vi "TestDigitizer.vi"() -> ()   [LabVIEW 2018]
uses:
  <extravilib>/ChannelInstances/Tag-c(t'DigitizerInfo.ctl',bool).lvlib
  <vilib>/userdefined/High Color/nirio_resource_hc.ctl
  D:/HardwareRevamp/AcustoXv2/Controls/DigitizerInfo.ctl
panel:
  in  "Digitizer ID":tag
  out "TIS Configured?":bool
  out "Clocking Option Configured?":bool
  out "Default Configured?":bool
  in  "Trigger Type":enum8{"Software", "Data Edge"}(ring)
  in  "Record Size (Samples)":u32=1024
  in  "Trigger Level (V)":dbl
  in  "Delay after Trigger (us)":dbl
  in  "Sampling Rate (Fs)":dbl=400000000.0 format="%#_6p"
  in  "Setup Digitizer":bool
  out "Digitizer Configured?":bool
  out "Digitizer Info":T1
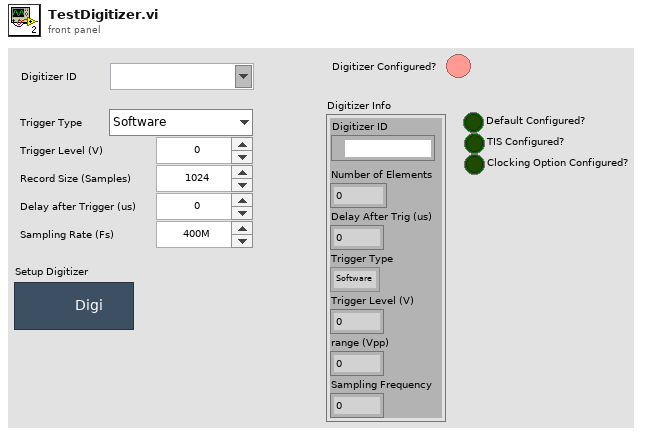
[diagram p1: front panel]
types:
  T1 = typedef "DigitizerInfo.ctl" = cluster{"Digitizer ID":T2, "Number of Elements":u16, "Delay After Trig (us)":dbl, "Trigger Type":enum8{"Software", "Data Edge"}, "Trigger Level (V)":dbl, "range (Vpp)":dbl, "Sampling Frequency":dbl}
  T2 = typedef "nirio_resource_hc.ctl" = tag
  T3 = typedef "Tag-c(t'DigitizerInfo.ctl',bool).lvlib/))Channel.ctl" = refnum<queue>
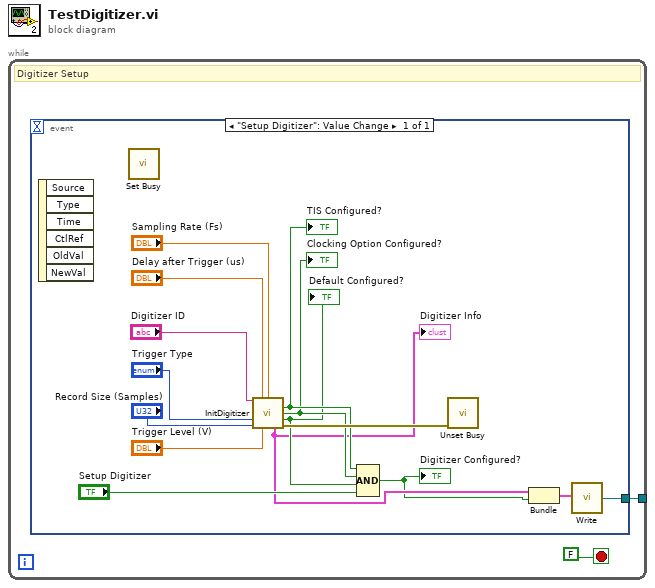
[diagram p0: block diagram]
diagram:
  n1 = while {
    tunnel: [w1] -> _
    stop <- FALSE stop-if-true
    # "Digitizer Setup"
    n2 = event shown="[0] \"Setup Digitizer\": Value Change" {
      selector: _ -> [_]
      dyn-events: _ -> [_]
      timeout: _ -> [_]
      tunnel: [w6] -> w1
      event "Setup Digitizer": Value Change {
        n3 = event-data() -> ()  [unwired: 1 in, 6 out]
        n4 = call <vilib>:"Set Busy.vi"() -> ()  [unwired: 10 in, 2 out]
        n5 = call "InitDigitizer.vi"("Digitizer ID"="Digitizer ID", "Delay After Trig (us)"="Delay after Trigger (us)", "Sampling Frequency"="Sampling Rate (Fs)", "Trigger Type"="Trigger Type", "Record Size"="Record Size (Samples)", "Trigger Level (V)"="Trigger Level (V)") -> ("TIS Configured?"=w15:bool, "Clocking Configured?"=w14:bool, "Default Configured?"=w13:bool, "Digitizer Info"=w4:T1, "Error out"=w16:errorcluster)  [unwired: 5 in]
        "TIS Configured?" <- w15
        "Clocking Option Configured?" <- w14
        "Default Configured?" <- w13
        "Digitizer Info" <- w4
        n6 = Compound Arithmetic op=AND(w15, w14, w13, "Setup Digitizer") -> (w3:bool)
        "Digitizer Configured?" <- w3
        n7 = call <vilib>:"Unset Busy.vi"("error in (no error)"=w16) -> ()  [unwired: 10 in, 1 out]
        n8 = Bundle("Digitizer Info"=w4, w3) -> (w5:cluster{"Digitizer Info":T1, bool})  [unwired: 1 in]
        n9 = call <extravilib>:"Write.vi"("element"=w5) -> ("channel"=w6:T3)  [unwired: 1 out]
      }
    }
  }
